vi "WinchMotor.vi"   [LabVIEW 2012]
uses:
  State_Machine_Enum.ctl
  Robot Global Data.vi
types:
  T1 = typedef "State_Machine_Enum.ctl" = enum16{"Init", "Idle", "Start", "Do", "Stop"}
  T2 = typedef "WPI_MotorControlDeviceRef.ctl" = cluster{"DeviceStatus":errorcluster, "Type":enum16{"PWM", "CAN"}, "PWM":cluster{"Digital Module":T3, "PWM Channel":T4, "DeadBand":T5}, "CAN":cluster{"Device Number":u8, "Control Mode":T6, "Semaphore":T7, "Max Vout":dbl}, "Invert":bool, "TransformRef":T8, "InvTransformRef":T8}
  T3 = typedef "FPGA_TypedefDigitalModule.ctl" = enum16{"Digital Module 1", "Digital Module 2"}
  T4 = typedef "FPGA_DIOPWMChannel.ctl" = enum8{"PWM 1", "PWM 2", "PWM 3", "PWM 4", "PWM 5", "PWM 6", "PWM 7", "PWM 8", "PWM 9", "PWM 10", "Invalid"}
  T5 = typedef "WPI_PWMDeadband.ctl" = cluster{"Name":string, "maxPositivePwm":i32, "minPositivePwm":i32, "centerPwm":i32, "maxNegativePwm":i32, "minNegativePwm":i32, "angularRange":u16}
  T6 = typedef "WPI_CANJaguar_ControlMode.ctl" = enum8{"Percent VBus", "Current", "Speed", "Position", "Voltage"}
  T7 = typedef "Semaphore RefNum" = refnum<k1>
  T8 = typedef "WPI_PWMTransform_ConPane.ctl" = refnum<vi>
  T9 = typedef "WPI_DigitalInputDevRef.ctl" = cluster{"DevStatus":errorcluster, "DIO Channel":T10, "Digital Module":T3}
  T10 = typedef "FPGA_DIOChannel.ctl" = enum8{"DIO 1", "DIO 2", "DIO 3", "DIO 4", "DIO 5", "DIO 6", "DIO 7", "DIO 8", "DIO 9", "DIO 10", "DIO 11", "DIO 12", "DIO 13", "DIO 14", "Invalid"}
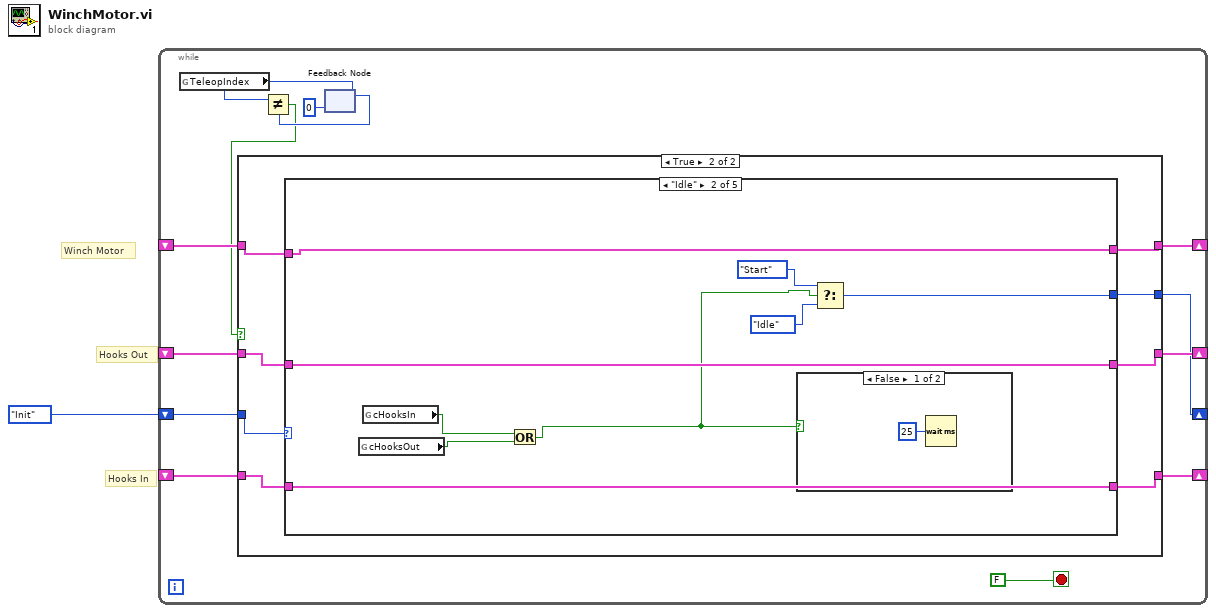
[diagram p0: block diagram]
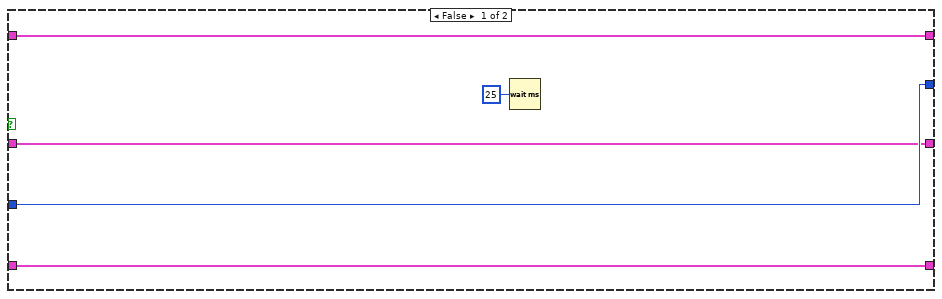
[diagram p2: hidden frame]
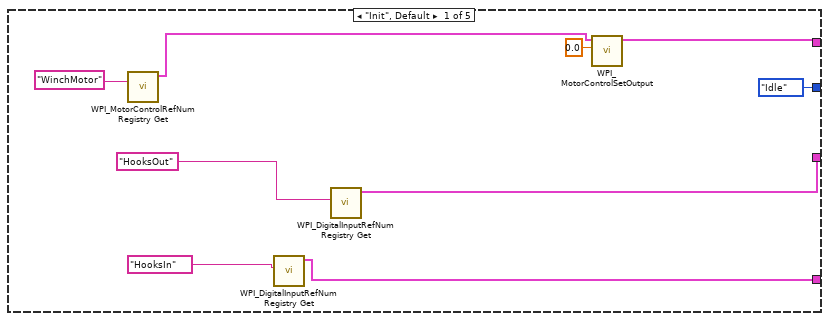
[diagram p3: hidden frame]
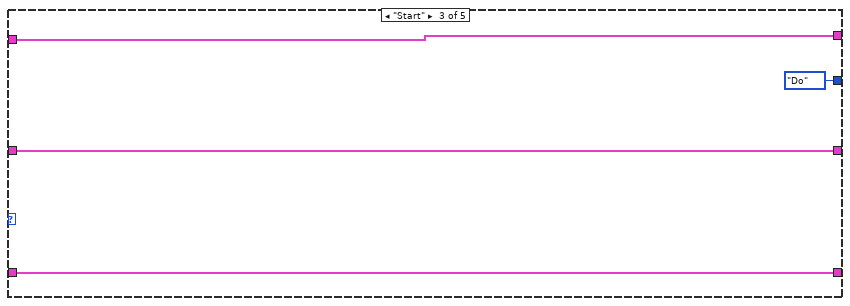
[diagram p5: hidden frame]
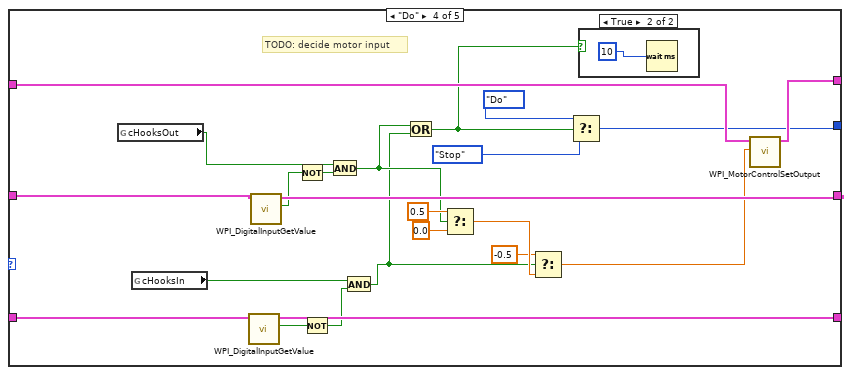
[diagram p6: hidden frame]
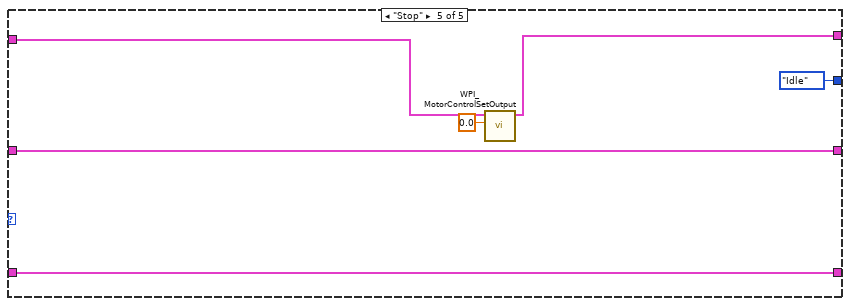
[diagram p8: hidden frame]
diagram:
  # "Hooks In"
  # "Hooks Out"
  # "Winch Motor"
  n1 = while {
    shift-right: [w12] -> _
    shift-left: _ -> [w13]
    shift-right: [w11] -> _
    shift-left: _ -> [w8]
    shift-right: [w10] -> _
    shift-left: _ -> [w9]
    shift-right: [w6] -> _
    shift-left: State_Machine_Enum."Init" ("State") -> [w7]
    stop <- FALSE stop-if-true
    n2 = global read "Robot Global Data.vi" "TeleopIndex"() -> (w4:i32)
    n3 = feedback #1(0 ("TeleopIndex")) -> (w5:i32)
    n4 = Not Equal?(x=w4, y=w5) -> (x != y?=w2:bool)
    n5 = case shown="True" w2 {
      tunnel: w13 -> [w19 w27]
      tunnel: [w19 w26] -> w12
      tunnel: [w17 w25] -> w11
      tunnel: [w16 w24] -> w10
      tunnel: w9 -> [w16 w23]
      tunnel: w8 -> [w17 w22]
      tunnel: w7 -> [w18 w21]
      tunnel: [w18 w20] -> w6
      frame False {
        n6 = Wait (ms)(milliseconds to wait=u32 25) -> ()  [unwired: 1 out]
      }
      frame True {
        n7 = case shown="\"Idle\"" w21 {
          tunnel: w27 -> [_ w37 w49 w73 w77]
          tunnel: [w29 w37 w49 w72 w76] -> w26
          tunnel: [w33 w44 w48 w71 w79] -> w25
          tunnel: [w32 w43 w47 w70 w78] -> w24
          tunnel: w23 -> [_ w43 w47 w69 w78]
          tunnel: w22 -> [_ w44 w48 w68 w79]
          tunnel: [State_Machine_Enum."Idle" ("State") w45 State_Machine_Enum."Do" ("f") w65 State_Machine_Enum."Idle" ("State")] -> w20
          frame "Init", Default {
            n8 = call <vilib>:"WPI_MotorControlRefNum Registry Get.vi"("refnum name"="WinchMotor") -> ("MotorControlDevRef"=w28:T2)  [unwired: 9 in, 1 out]
            n9 = call <vilib>:"WPI_DigitalInputRefNum Registry Get.vi"("refnum name"="HooksIn") -> ("DigitalInputDevRef"=w32:T9)  [unwired: 9 in, 1 out]
            n10 = call <vilib>:"WPI_DigitalInputRefNum Registry Get.vi"("refnum name"="HooksOut") -> ("DigitalInputDevRef"=w33:T9)  [unwired: 9 in, 1 out]
            n11 = call <vilib>:"WPI_MotorControlSetOutput.vi"("Output"=0.0, "MotorControlDevRef"=w28) -> ("MotorControlDevRef"=w29:T2)  [unwired: 7 in, 2 out]
          }
          frame "Idle" {
            n12 = global read "Robot Global Data.vi" "cHooksOut"() -> (w41:bool)
            n13 = global read "Robot Global Data.vi" "cHooksIn"() -> (w42:bool)
            n14 = Or(x=w42, y=w41) -> (x .or. y?=w40:bool)
            n15 = case shown="False" w40 {
              frame False {
                n16 = Wait (ms)(milliseconds to wait=u32 25) -> ()  [unwired: 1 out]
              }
              frame True {
              }
            }
            n17 = Select(t=State_Machine_Enum."Start" ("f"), s=w40, f=State_Machine_Enum."Idle") -> (s? t:f=w45:T1)
          }
          frame "Start" {
          }
          frame "Do" {
            # "TODO: decide motor input"
            n18 = global read "Robot Global Data.vi" "cHooksOut"() -> (w61:bool)
            n19 = global read "Robot Global Data.vi" "cHooksIn"() -> (w62:bool)
            n20 = call <vilib>:"WPI_DigitalInputGetValue.vi"("DigitalInputDevRef"=w69) -> ("Value"=w64:bool, "DigitalInputDevRef"=w70:T9)  [unwired: 8 in, 1 out]
            n21 = call <vilib>:"WPI_DigitalInputGetValue.vi"("DigitalInputDevRef"=w68) -> ("Value"=w60:bool, "DigitalInputDevRef"=w71:T9)  [unwired: 8 in, 1 out]
            n22 = Not(x=w60) -> (.not. x?=w59:bool)
            n23 = Not(x=w64) -> (.not. x?=w63:bool)
            n24 = And(x=w61, y=w59) -> (x .and. y?=w53:bool)
            n25 = And(x=w62, y=w63) -> (x .and. y?=w52:bool)
            n26 = Or(x=w53, y=w52) -> (x .or. y?=w51:bool)
            n27 = Select(t=0.5, s=w53, f=0.0) -> (s? t:f=w57:dbl)
            n28 = Select(t=-0.5, s=w52, f=w57) -> (s? t:f=w54:dbl)
            n29 = Select(t=State_Machine_Enum."Do" ("State"), s=w51, f=State_Machine_Enum."Stop" ("State")) -> (s? t:f=w65:T1)
            n30 = case shown="True" w51 {
              frame False {
              }
              frame True {
                n31 = Wait (ms)(milliseconds to wait=u32 10) -> ()  [unwired: 1 out]
              }
            }
            n32 = call <vilib>:"WPI_MotorControlSetOutput.vi"("Output"=w54, "MotorControlDevRef"=w73) -> ("MotorControlDevRef"=w72:T2)  [unwired: 7 in, 2 out]
          }
          frame "Stop" {
            n33 = call <vilib>:"WPI_MotorControlSetOutput.vi"("Output"=0.0, "MotorControlDevRef"=w77) -> ("MotorControlDevRef"=w76:T2)  [unwired: 7 in, 2 out]
          }
        }
      }
    }
    n34 = feedback-in #1(w4) -> ()
  }
